vi "Leitura_pressão_temperatura.vi"() -> ()   [LabVIEW 2019]
uses:
  <vilib>/Analysis/NI_AALBase.lvlib
panel:
  out "Error out":errorcluster {"code" format="%.0x"}
  out "Valvula Suc":sgl
  in  "Sub Index":u8 format="%.0x"
  in  "Index":u16=4104 format="%.0x"
  out "error out":errorcluster
  out "XY Graph 2":cluster{dbl[], dbl[]}[](graph)
  out "Stop Press":bool
  out "Stop Temp":bool
  in  "stop":bool
  out "Zerar Temp":bool
  out "Zerar Press":bool
  in  "Zerar":bool
  out "Corpo [ºC]":dbl
  out "Descarga [ºC]":dbl
  out "Reservatório [ºC]":dbl
  out "Sucção [ºC]":dbl
  out "Intermed":dbl format="%0.4f"
  out "Descarga A0":dbl format="%0.4f"
  out "Sucção A1":dbl format="%0.4f"
  out "XY Graph":cluster{dbl[], dbl[]}[](graph)
  out "Descarga/Sucção":dbl
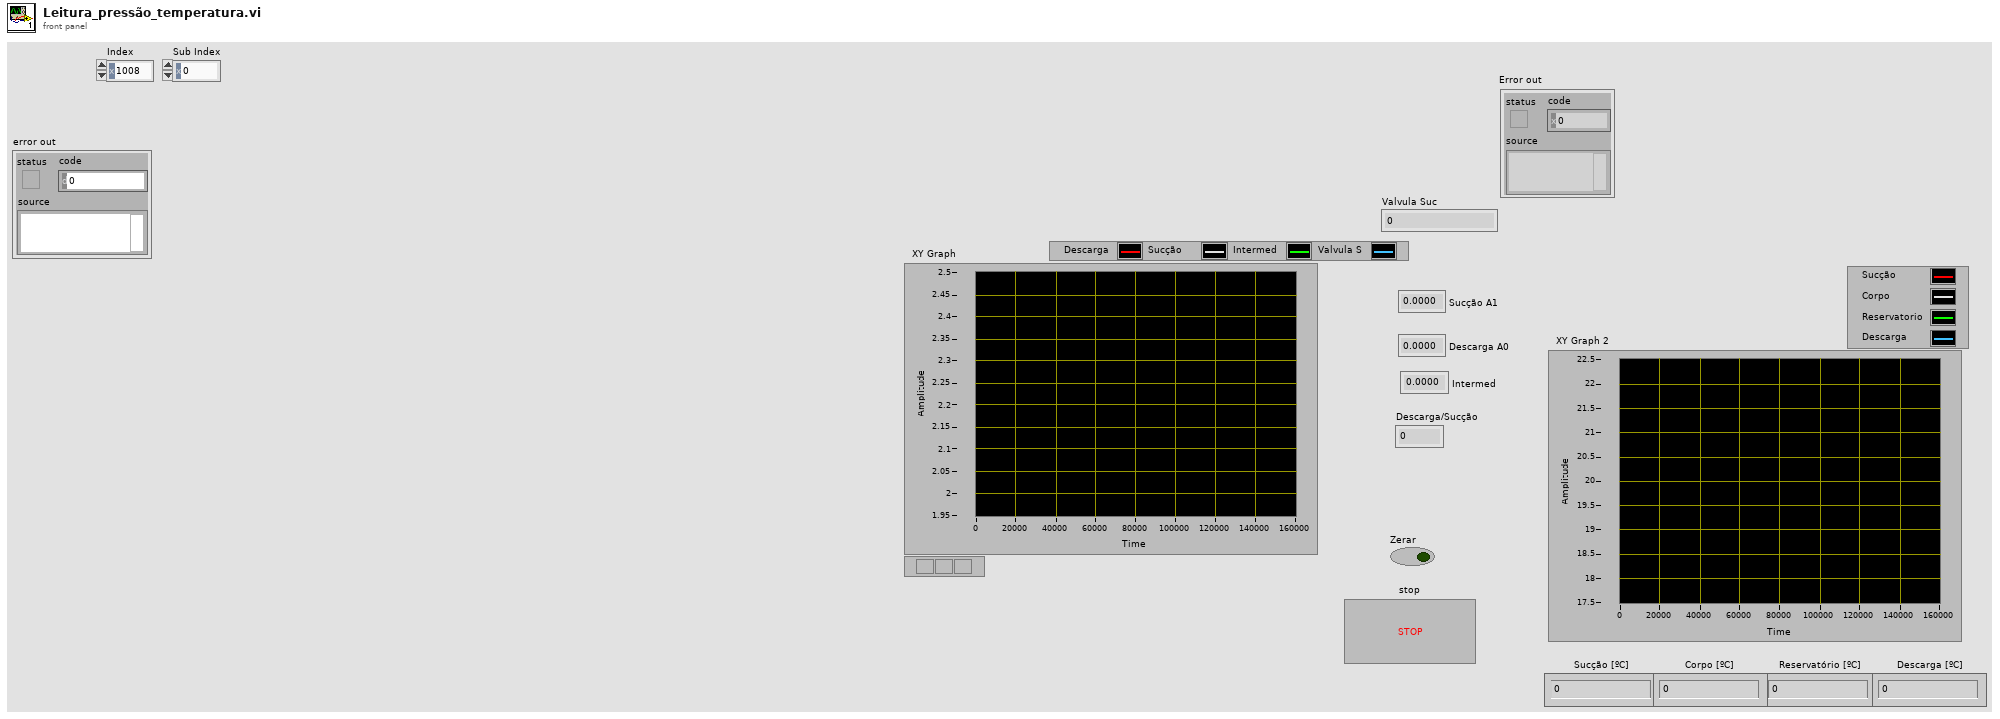
[diagram p1: front panel]
types:
  T1 = enum16{"start remote node", "stop remote node", "reset node", "reset communication", "enter preoperational"}
  T2 = typedef "xobjhandle.ctl" = u32
  T3 = enum16{"big-endian, network order", "native, host order", "little-endian"}
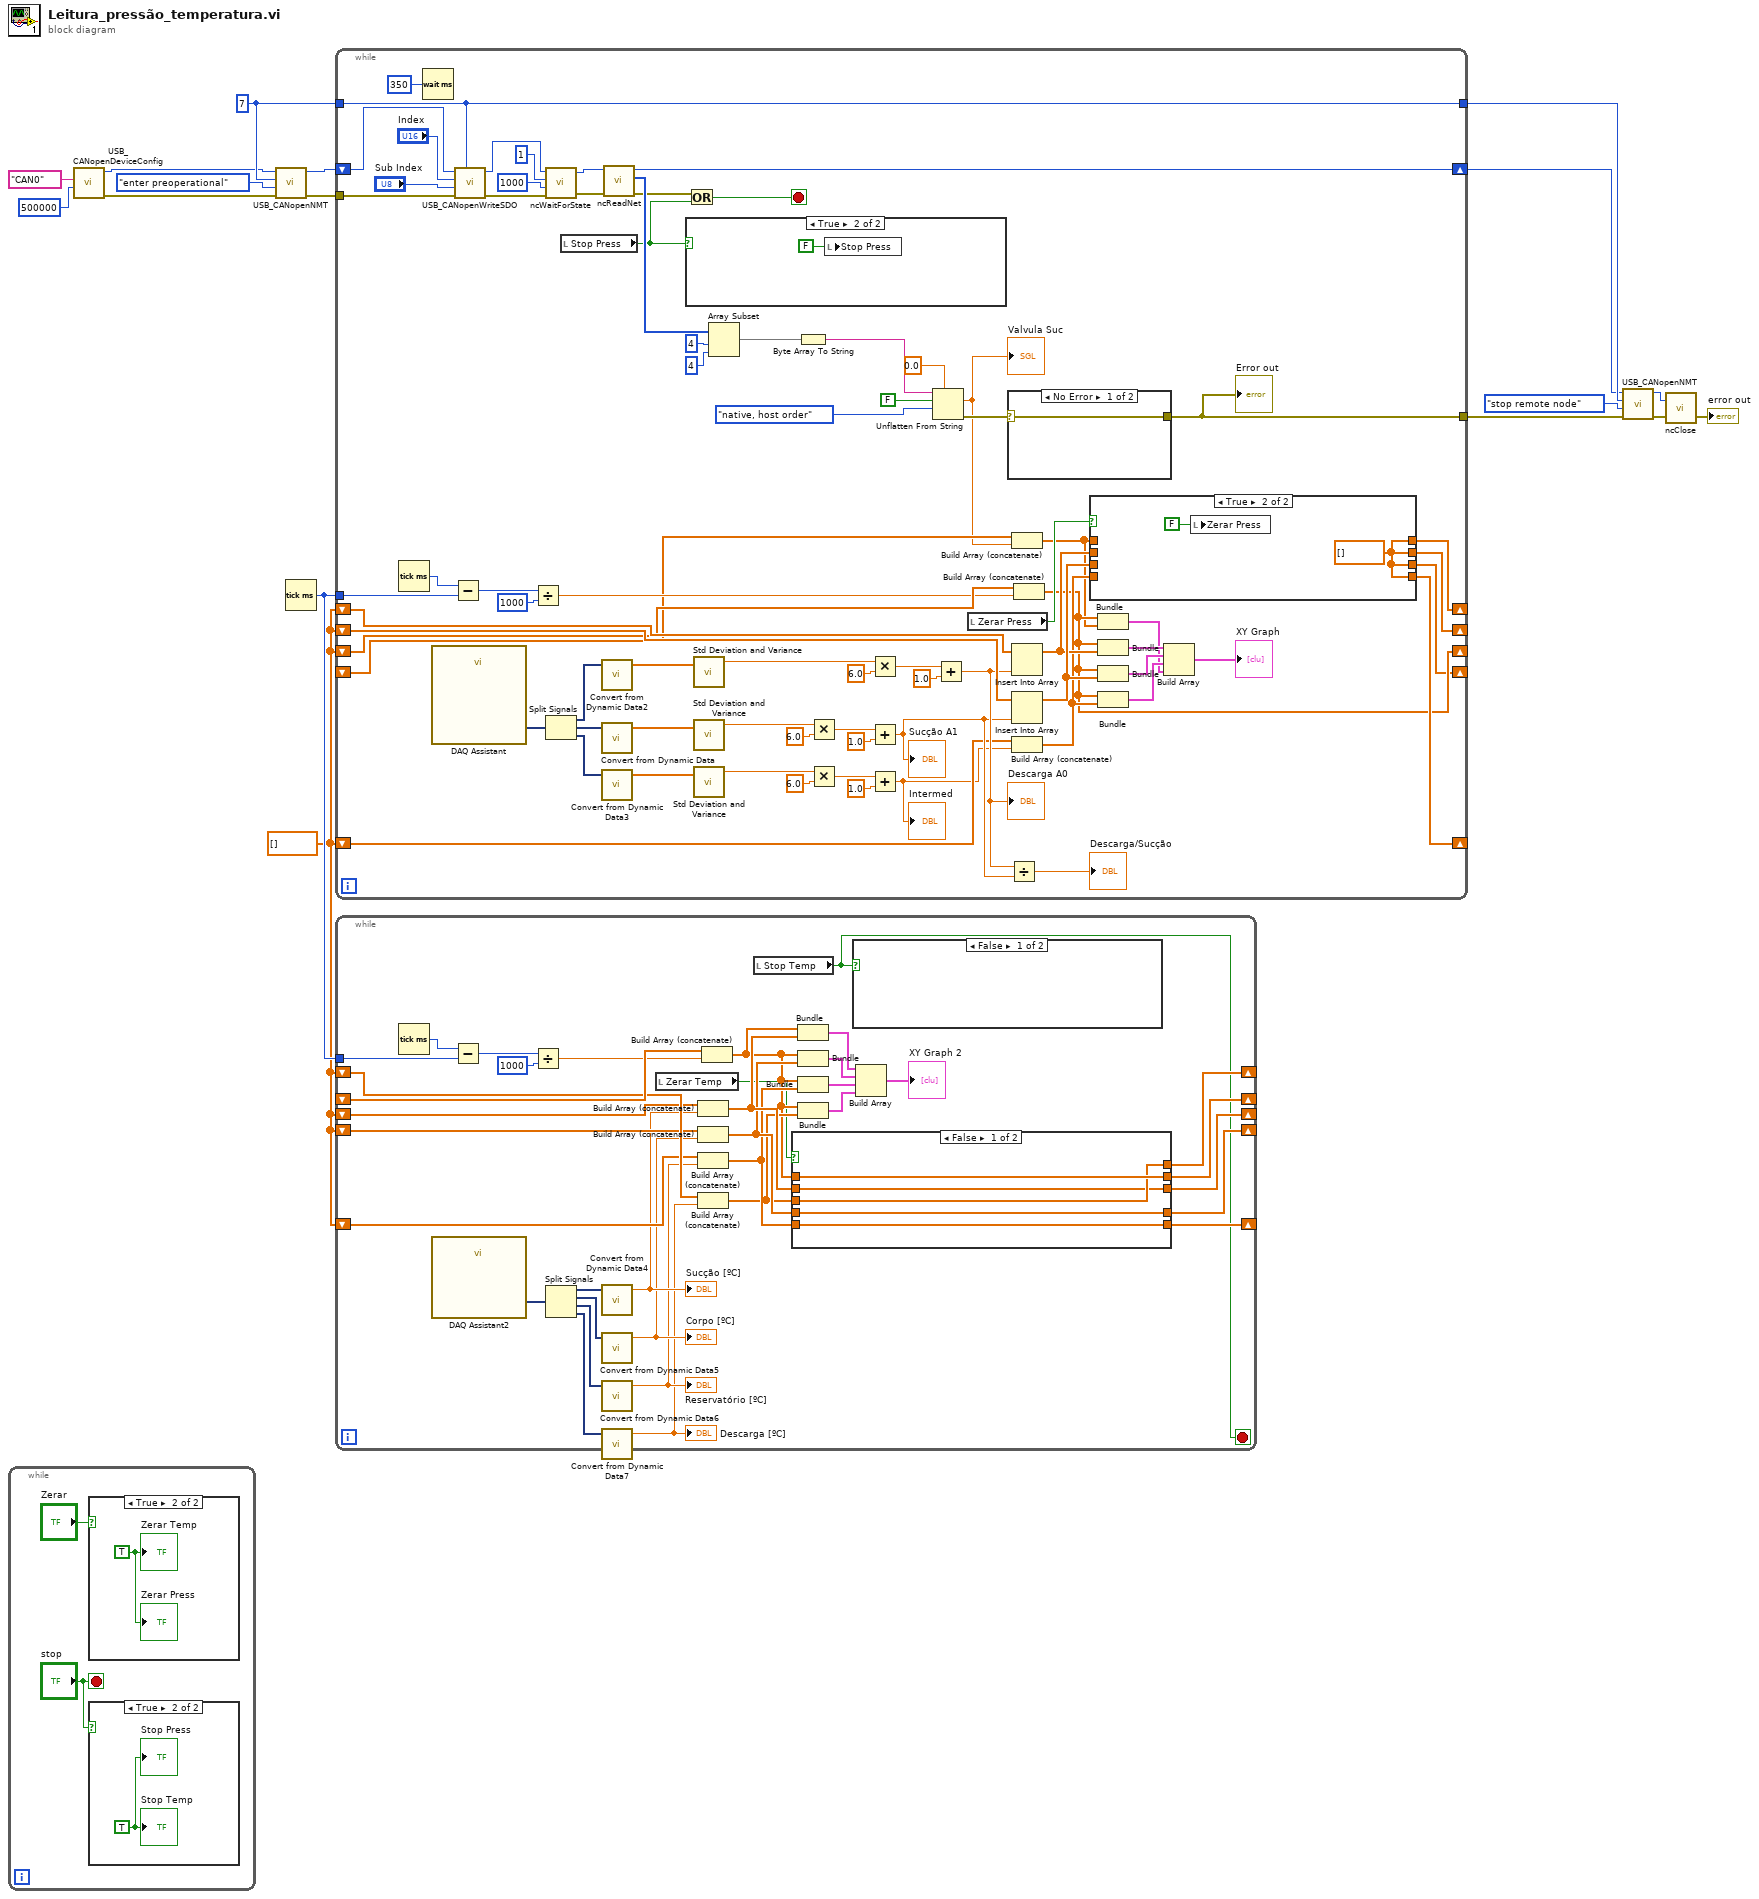
[diagram p0: block diagram]
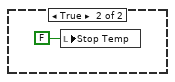
[diagram p4: hidden frame]
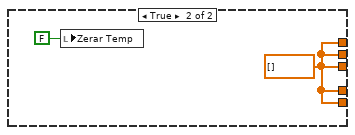
[diagram p5: hidden frame]
diagram:
  w8 = u32 7 ("milliseconds to wait")
  w16 = dbl[] []
  n1 = while {
    stop <- "stop" stop-if-true
    n2 = case shown="True" "Zerar" {
      frame False {
      }
      frame True {
        w21 = TRUE
        "Zerar Press" <- w21
        "Zerar Temp" <- w21
      }
    }
    n3 = case shown="True" "stop" {
      frame False {
      }
      frame True {
        w20 = TRUE
        "Stop Press" <- w20
        "Stop Temp" <- w20
      }
    }
  }
  n4 = call "USB_CANopenDeviceConfig.vi"("Baudrate"=u32 500000, "Interface"="CAN0") -> ("Error out"=w5:errorcluster, "ObjHandle out"=w3:T2)  [unwired: 8 in]
  n5 = call "USB_CANopenNMT.vi"("error in"=w5, "Mode"=T1."enter preoperational", "Node ID"=w8, "ObjHandle in"=w3) -> ("error out"=w2:errorcluster, "ObjHandle out"=w1:T2)  [unwired: 2 in]
  n6 = Tick Count (ms)() -> (millisecond timer value=w17:u32)
  n7 = while {
    shift-right: [w83] -> _
    shift-left: w16 -> [w91]
    shift-right: [w84] -> _
    shift-left: w16 -> [w90]
    shift-right: [w25] -> _
    shift-left: w16 -> [w74]
    tunnel: w17 -> [w65]
    shift-right: [w54] -> _
    shift-left: w16 -> [w57]
    tunnel: [w37] -> w12
    tunnel: [w40] -> w10
    tunnel: w8 -> [w40]
    shift-right: [w39] -> w9
    shift-left: w1 -> [w29]
    tunnel: w2 -> [w28]
    shift-right: [w22] -> _
    shift-left: _ -> [w27]
    stop <- w42 stop-if-true
    n8 = Tick Count (ms)() -> (millisecond timer value=w67:u32)
    n9 = Wait (ms)(milliseconds to wait=u32 350) -> ()  [unwired: 1 out]
    n10 = call "DAQ Assistant"() -> ("data"=w96:dynamicdata)  [unwired: 17 in, 2 out]
    n11 = Subtract(x=w67, y=w65) -> (x-y=w66:u32)
    n12 = call "USB_CANopenWriteSDO.vi"("Node ID"=w40, "error in"=w28, "Sub Index"="Sub Index", "Index"="Index", "ObjHandle in"=w29) -> ("error out"=w31:errorcluster, "ObjHandle out"=w33:T2)  [unwired: 5 in]
    n13 = Divide(x=w66, y=u32 1000) -> (x/y=w68:dbl)
    n14 = call <vilib>:"ncWaitForState.vi"("Error in"=w31, "Timeout"=u32 1000, "DesiredState"=u32 1, "ObjHandle in"=w33) -> ("Error out"=w30:errorcluster, "ObjHandle out"=w32:T2)  [unwired: 1 out]
    n15 = Split Signals(w96) -> (w94:dynamicdata, w95:dynamicdata, w64:dynamicdata)  [unwired: 3 in]
    n16 = local read "Stop Press"() -> (w41:bool)
    n17 = call "Convert from Dynamic Data2"("Dynamic Data Type"=w94) -> ("Array"=w93:dbl[])  [unwired: 3 in]
    n18 = call "Convert from Dynamic Data"("Dynamic Data Type"=w95) -> ("Array"=w92:dbl[])  [unwired: 3 in]
    n19 = call "Convert from Dynamic Data3"("Dynamic Data Type"=w64) -> ("Array"=w63:dbl[])  [unwired: 3 in]
    n20 = call <vilib>:"ncReadNet.vi"("ObjHandle in"=w32, "Error in"=w30) -> ("ObjHandle out"=w39:T2, "Data"=w43:u8[], "Error out"=w36:errorcluster)  [unwired: 2 in, 4 out]
    n21 = case shown="True" w41 {
      frame False {
      }
      frame True {
        n22 = local write "Stop Press"(FALSE ("Stop Press")) -> ()
      }
    }
    n23 = Or(x=w36, y=w41) -> (x .or. y?=w42:bool)
    n24 = call <vilib>:"Std Deviation and Variance.vi"("X"=w93) -> ("mean"=w88:dbl)  [unwired: 1 in, 2 out]
    n25 = call <vilib>:"Std Deviation and Variance.vi"("X"=w92) -> ("mean"=w86:dbl)  [unwired: 1 in, 2 out]
    n26 = call <vilib>:"Std Deviation and Variance.vi"("X"=w63) -> ("mean"=w59:dbl)  [unwired: 1 in, 2 out]
    n27 = Array Subset(array=w43, index=4, length=4) -> (w45:u8[])
    n28 = Byte Array To String(unsigned byte array=w45) -> (string=w52:string)
    n29 = Multiply(x=w86, y=6.0) -> (x*y=w80:dbl)
    n30 = Multiply(x=w59, y=6.0) -> (x*y=w62:dbl)
    n31 = Multiply(x=w88, y=6.0) -> (x*y=w79:dbl)
    n32 = Add(x=w80, y=1.0) -> (x+y=w75:dbl)
    "Sucção A1" <- w75
    n33 = Add(x=w62, y=1.0) -> (x+y=w56:dbl)
    "Intermed" <- w56
    n34 = Unflatten From String(type=sgl 0.0, binary string=w52, data includes array or string size? (T)=FALSE, byte order (0:big-endian, network order)=T3."native, host order") -> (value=w26:sgl, error out=w38:errorcluster)  [unwired: 1 in, 1 out]
    "Valvula Suc" <- w26
    n35 = Add(x=w79, y=1.0) -> (x+y=w76:dbl)
    "Descarga A0" <- w76
    n36 = local read "Zerar Press"() -> (w53:bool)
    n37 = case shown="No Error" w38 {
      selector: w38 -> [w97 _]
      tunnel: [w97 _] -> w37
      frame No Error {
      }
      frame Error {
      }
    }
    "Error out" <- w37
    n38 = Divide(x=w76, y=w75) -> (x/y=→"Descarga/Sucção":dbl)
    n39 = Build Array (concatenate)(w27, w26) -> (w23:dbl[])
    n40 = Insert Into Array(array=w91, new element=w76) -> (w72:dbl[])  [unwired: 1 in]
    n41 = Insert Into Array(array=w90, new element=w75) -> (w73:dbl[])  [unwired: 1 in]
    n42 = Build Array (concatenate)(w57, w56) -> (w55:dbl[])
    n43 = Build Array (concatenate)(w74, w68) -> (w25:dbl[])
    n44 = case shown="True" w53 {
      tunnel: w73 -> [w102 _]
      tunnel: [w102 w103] -> w84
      tunnel: w72 -> [w101 _]
      tunnel: [w101 w103] -> w83
      tunnel: w55 -> [w100 _]
      tunnel: [w100 w103] -> w54
      tunnel: w23 -> [w99 _]
      tunnel: [w99 w103] -> w22
      frame False {
      }
      frame True {
        w103 = dbl[] []
        n45 = local write "Zerar Press"(FALSE ("Zerar Temp")) -> ()
      }
    }
    n46 = Bundle(w25, w23) -> (w24:cluster{dbl[], dbl[]})  [unwired: 1 in]
    n47 = Bundle(w25, w72) -> (w71:cluster{dbl[], dbl[]})  [unwired: 1 in]
    n48 = Bundle(w25, w73) -> (w70:cluster{dbl[], dbl[]})  [unwired: 1 in]
    n49 = Bundle(w25, w55) -> (w58:cluster{dbl[], dbl[]})  [unwired: 1 in]
    n50 = Build Array(w71, w70, w58, w24) -> (→"XY Graph":cluster{dbl[], dbl[]}[])
  }
  n51 = while {
    tunnel: w17 -> [w133]
    shift-right: [w122] -> _
    shift-left: w16 -> [w121]
    shift-right: [w124] -> _
    shift-left: w16 -> [w123]
    shift-right: [w126] -> _
    shift-left: w16 -> [w125]
    shift-right: [w128] -> _
    shift-left: w16 -> [w127]
    shift-right: [w129] -> _
    shift-left: _ -> [w131]
    stop <- w110 stop-if-true
    n52 = Tick Count (ms)() -> (millisecond timer value=w134:u32)
    n53 = call "DAQ Assistant2"() -> ("data"=w140:dynamicdata)  [unwired: 17 in, 2 out]
    n54 = Subtract(x=w134, y=w133) -> (x-y=w135:u32)
    n55 = Divide(x=w135, y=u32 1000) -> (x/y=w130:dbl)
    n56 = Split Signals(w140) -> (w139:dynamicdata, w138:dynamicdata, w137:dynamicdata, w136:dynamicdata)  [unwired: 4 in]
    n57 = call "Convert from Dynamic Data4"("Dynamic Data Type"=w139) -> ("Scalar"=w120:dbl)  [unwired: 3 in]
    "Sucção [ºC]" <- w120
    n58 = call "Convert from Dynamic Data5"("Dynamic Data Type"=w138) -> ("Scalar"=w119:dbl)  [unwired: 3 in]
    "Corpo [ºC]" <- w119
    n59 = call "Convert from Dynamic Data6"("Dynamic Data Type"=w137) -> ("Scalar"=w118:dbl)  [unwired: 3 in]
    "Reservatório [ºC]" <- w118
    n60 = call "Convert from Dynamic Data7"("Dynamic Data Type"=w136) -> ("Scalar"=w117:dbl)  [unwired: 3 in]
    "Descarga [ºC]" <- w117
    n61 = local read "Zerar Temp"() -> (w111:bool)
    n62 = Build Array (concatenate)(w121, w120) -> (w116:dbl[])
    n63 = Build Array (concatenate)(w123, w119) -> (w115:dbl[])
    n64 = Build Array (concatenate)(w125, w118) -> (w114:dbl[])
    n65 = Build Array (concatenate)(w127, w117) -> (w113:dbl[])
    n66 = Build Array (concatenate)(w131, w130) -> (w112:dbl[])
    n67 = local read "Stop Temp"() -> (w110:bool)
    n68 = case shown="False" w111 {
      tunnel: w112 -> [w146 _]
      tunnel: [w146 w147] -> w129
      tunnel: w113 -> [w145 _]
      tunnel: [w145 w147] -> w128
      tunnel: w114 -> [w144 _]
      tunnel: [w144 w147] -> w126
      tunnel: w115 -> [w143 _]
      tunnel: [w143 w147] -> w124
      tunnel: w116 -> [w142 _]
      tunnel: [w142 w147] -> w122
      frame False {
      }
      frame True {
        w147 = dbl[] []
        n69 = local write "Zerar Temp"(FALSE ("Zerar Temp")) -> ()
      }
    }
    n70 = Bundle(w112, w116) -> (w108:cluster{dbl[], dbl[]})  [unwired: 1 in]
    n71 = Bundle(w112, w115) -> (w107:cluster{dbl[], dbl[]})  [unwired: 1 in]
    n72 = Bundle(w112, w114) -> (w106:cluster{dbl[], dbl[]})  [unwired: 1 in]
    n73 = Bundle(w112, w113) -> (w105:cluster{dbl[], dbl[]})  [unwired: 1 in]
    n74 = case shown="False" w110 {
      frame False {
      }
      frame True {
        n75 = local write "Stop Temp"(FALSE ("Stop Temp")) -> ()
      }
    }
    n76 = Build Array(w108, w107, w106, w105) -> (→"XY Graph 2":cluster{dbl[], dbl[]}[])
  }
  n77 = call "USB_CANopenNMT.vi"("error in"=w12, "Mode"=T1."stop remote node", "Node ID"=w10, "ObjHandle in"=w9) -> ("error out"=w13:errorcluster, "ObjHandle out"=w15:T2)  [unwired: 2 in]
  n78 = call <vilib>:"ncClose.vi"("Error in"=w13, "ObjHandle in"=w15) -> ("Error out"=→"error out":errorcluster)  [unwired: 1 in]
